vi "LAInit.vi"(8 "Error Input":errorcluster caption="Error In", 10 "ApiKey":string, 11 "BaseUrl":string) -> (0 "Error Output":errorcluster caption="Error Out", 2 "Version":string, 3 "LiteAgent":T1)   [LabVIEW 2017, in "LiteAgentSDK.lvlib"]
uses:
  LiteAgentSDK.lvlib
  C:/Users/Jan/Projects/LiteAgentSDK-LabVIEW/Source/Bin/LiteAgentSDK.LabVIEW.dll
  Bin/LiteAgentSDK.LabVIEW.dll
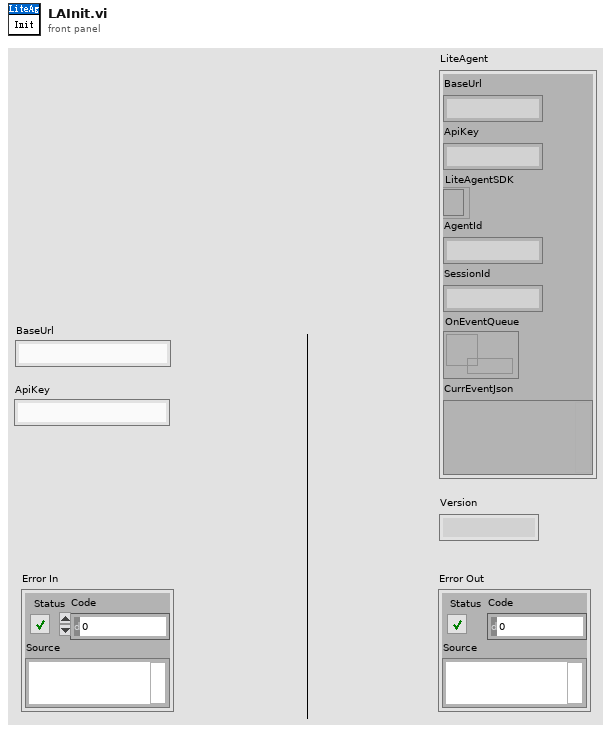
[diagram p1: front panel]
types:
  T1 = cluster{"BaseUrl":string, "ApiKey":string, "LiteAgentSDK":refnum<k24>, "AgentId":string, "SessionId":string, "OnEventQueue":refnum<queue>, "CurrEventJson":variant}
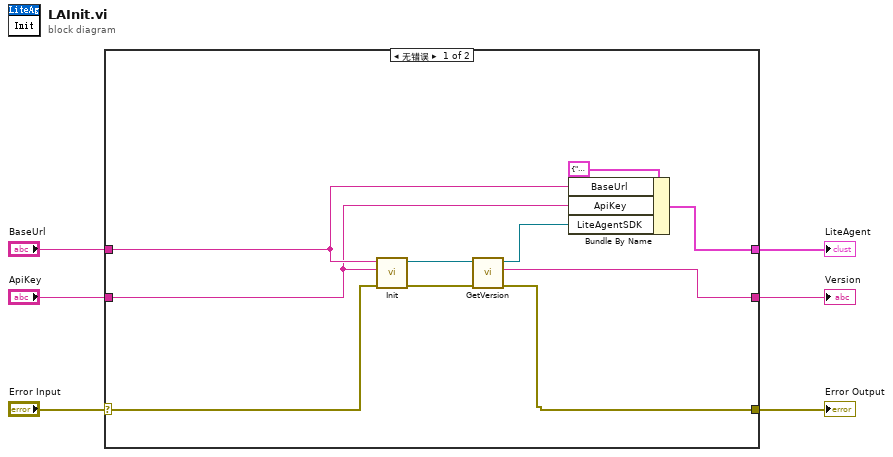
[diagram p0: block diagram]
diagram:
  n1 = case shown="无错误" "Error Input" {
    selector: "Error Input" -> [w16 w17]
    tunnel: [w9 w17] -> w5
    tunnel: "BaseUrl" -> [w14 _]
    tunnel: "ApiKey" -> [w13 _]
    tunnel: [w15 _] -> w2
    tunnel: [w7 _] -> w1
    frame No Error {
      n2 = call "Init.vi"("Error Input"=w16, "ApiKey"=w13, "BaseUrl"=w14) -> ("Error Output"=w10:errorcluster, "LiteAgentSDK Output"=w11:refnum<k24>)  [unwired: 7 in]
      n3 = call "GetVersion.vi"("Error Input"=w10, "LiteAgentSDK Input"=w11) -> ("Error Output"=w9:errorcluster, "Version"=w7:string, "LiteAgentSDK Output"=w8:refnum<k24>)  [unwired: 7 in]
      n4 = Bundle By Name(cluster=T1 {"BaseUrl"="", "ApiKey"="", "LiteAgentSDK"=refnum, "AgentId"="", "SessionId"="", "OnEventQueue"=refnum, "CurrEventJson"=variant} ("LiteAgent"), "BaseUrl"=w14, "ApiKey"=w13, "LiteAgentSDK"=w8) -> (w15:T1)
    }
    frame Error {
    }
  }
  "Error Output" <- w5
  "LiteAgent" <- w2
  "Version" <- w1
